vi "MapColor_makeRamp.vi"(1 "ColorMap\narray IN":u32[](array[numeric])=[0, 196608, 393216, 589824, 786432, 983040, 1179648, 1376256, 1572864, 1769472, 1966080, 2162688, 2359296, 2555904, 2752512, 2949120, 3145728, 3342336, 3538944, 3735552, 3932160, 4128768, 4325376, 4521984, 4718592, 4915200, 5111808, 5308416, 5505024, 5701632, 5898240, 6094848, 6291456, 6488064, 6684672, 6881280, 7077888, 7274496, 7471104, 7667712, 7864320, 8060928, 8257536, 8454144, 8650752, 8847360, 9043968, 9240576, 9437184, 9633792, 9830400, 10027008, 10223616, 10420224, 10616832, 10813440, 11010048, 11206656, 11403264, 11599872, 11796480, 11993088, 12189696, 12386304, 12582912, 12779520, 12976128, 13172736, 13369344, 13565952, 13762560, 13959168, 14155776, 14352384, 14548992, 14745600, 14942208, 15138816, 15335424, 15532032, 15728640, 15925248, 16121856, 16318464, 16515072, 16711680, 16712448, 16713216, 16713984, 16714752, 16715520, 16716288, 16717056, 16717824, 16718592, 16719360, 16720128, 16720896, 16721664, 16722432, 16723200, 16723968, 16724736, 16725504, 16726272, 16727040, 16727808, 16728576, 16729344, 16730112, 16730880, 16731648, 16732416, 16733184, 16733952, 16734720, 16735488, 16736256, 16737024, 16737792, 16738560, 16739328, 16740096, 16740864, 16741632, 16742400, 16743168, 16743936, 16744704, 16745472, 16746240, 16747008, 16747776, 16748544, 16749312, 16750080, 16750848, 16751616, 16752384, 16753152, 16753920, 16754688, 16755456, 16756224, 16756992, 16757760, 16758528, 16759296, 16760064, 16760832, 16761600, 16762368, 16763136, 16763904, 16764672, 16765440, 16766208, 16766976, 16767744, 16768512, 16769280, 16770048, 16770816, 16771584, 16772352, 16773120, 16773888, 16774656, 16775424, 16776192, 16776960, 16776963, 16776966, 16776969, 16776972, 16776975, 16776977, 16776980, 16776983, 16776986, 16776989, 16776992, 16776995, 16776998, 16777001, 16777004, 16777007, 16777009, 16777012, 16777015, 16777018, 16777021, 16777024, 16777027, 16777030, 16777033, 16777036, 16777038, 16777041, 16777044, 16777047, 16777050, 16777053, 16777056, 16777059, 16777062, 16777065, 16777068, 16777070, 16777073, 16777076, 16777079, 16777082, 16777085, 16777088, 16777091, 16777094, 16777097, 16777100, 16777102, 16777105, 16777108, 16777111, 16777114, 16777117, 16777120, 16777123, 16777126, 16777129, 16777132, 16777134, 16777137, 16777140, 16777143, 16777146, 16777149, 16777152, 16777155, 16777158, 16777161, 16777163, 16777166, 16777169, 16777172, 16777175, 16777178, 16777181, 16777184, 16777187, 16777190, 16777193, 16777195, 16777198, 16777201, 16777204, 16777207]) -> (0 "ColorMap\narray OUT":u32[](array[numeric])=[0, 196608, 393216, 589824, 786432, 983040, 1179648, 1376256, 1572864, 1769472, 1966080, 2162688, 2359296, 2555904, 2752512, 2949120, 3145728, 3342336, 3538944, 3735552, 3932160, 4128768, 4325376, 4521984, 4718592, 4915200, 5111808, 5308416, 5505024, 5701632, 5898240, 6094848, 6291456, 6488064, 6684672, 6881280, 7077888, 7274496, 7471104, 7667712, 7864320, 8060928, 8257536, 8454144, 8650752, 8847360, 9043968, 9240576, 9437184, 9633792, 9830400, 10027008, 10223616, 10420224, 10616832, 10813440, 11010048, 11206656, 11403264, 11599872, 11796480, 11993088, 12189696, 12386304, 12582912, 12779520, 12976128, 13172736, 13369344, 13565952, 13762560, 13959168, 14155776, 14352384, 14548992, 14745600, 14942208, 15138816, 15335424, 15532032, 15728640, 15925248, 16121856, 16318464, 16515072, 16711680, 16712448, 16713216, 16713984, 16714752, 16715520, 16716288, 16717056, 16717824, 16718592, 16719360, 16720128, 16720896, 16721664, 16722432, 16723200, 16723968, 16724736, 16725504, 16726272, 16727040, 16727808, 16728576, 16729344, 16730112, 16730880, 16731648, 16732416, 16733184, 16733952, 16734720, 16735488, 16736256, 16737024, 16737792, 16738560, 16739328, 16740096, 16740864, 16741632, 16742400, 16743168, 16743936, 16744704, 16745472, 16746240, 16747008, 16747776, 16748544, 16749312, 16750080, 16750848, 16751616, 16752384, 16753152, 16753920, 16754688, 16755456, 16756224, 16756992, 16757760, 16758528, 16759296, 16760064, 16760832, 16761600, 16762368, 16763136, 16763904, 16764672, 16765440, 16766208, 16766976, 16767744, 16768512, 16769280, 16770048, 16770816, 16771584, 16772352, 16773120, 16773888, 16774656, 16775424, 16776192, 16776960, 16776963, 16776966, 16776969, 16776972, 16776975, 16776977, 16776980, 16776983, 16776986, 16776989, 16776992, 16776995, 16776998, 16777001, 16777004, 16777007, 16777009, 16777012, 16777015, 16777018, 16777021, 16777024, 16777027, 16777030, 16777033, 16777036, 16777038, 16777041, 16777044, 16777047, 16777050, 16777053, 16777056, 16777059, 16777062, 16777065, 16777068, 16777070, 16777073, 16777076, 16777079, 16777082, 16777085, 16777088, 16777091, 16777094, 16777097, 16777100, 16777102, 16777105, 16777108, 16777111, 16777114, 16777117, 16777120, 16777123, 16777126, 16777129, 16777132, 16777134, 16777137, 16777140, 16777143, 16777146, 16777149, 16777152, 16777155, 16777158, 16777161, 16777163, 16777166, 16777169, 16777172, 16777175, 16777178, 16777181, 16777184, 16777187, 16777190, 16777193, 16777195, 16777198, 16777201, 16777204, 16777207])   [LabVIEW 2010]
panel:
  in  "ColorMap\nring":u16(ring) caption="Standard Colormap" items=["", "Black-Red-Yellow-White"]
  in  "Cancel":bool
  in  "Accept":bool
  out "VI ref":refnum<vi>
  in  "close":bool
  in  "Scrollbar":i32(c297)=64
  out "ColorRamp":u32[](array[colorbox])=[180, 263349, 526518, 789687, 1052856, 1316026, 1579195, 1842364, 2105533, 2368702, 2631871, 2895040, 3158209, 3421378, 3684548, 3947717, 4145094, 4408263, 4671432, 4934601, 5197770, 5460939, 5724108, 5987278, 6250447, 6513616, 6776785, 7039954, 7303123, 7566292, 7829461, 8092630, 8355800, 8618969, 8882138, 9145307, 9408476, 9671645, 9934814, 10197983, 10461152, 10724322, 10987491, 11250660, 11513829, 11776998, 12040167, 12303336, 12500713, 12763882, 13027052, 13290221, 13553390, 13816559, 14079728, 14342897, 14606066, 14869235, 15132404, 15395574, 15658743, 15921912, 16185081, 16448250, 16448250, 16447222, 16446194, 16445166, 16444138, 16443110, 16442082, 16506590, 16505562, 16504534, 16503506, 16502478, 16501450, 16500422, 16499394, 16498366, 16497595, 16496567, 16495539, 16560047, 16559019, 16557991, 16556963, 16555935, 16554907, 16553879, 16552851, 16551823, 16550795, 16549767, 16548739, 16547711, 16612219, 16611191, 16610163, 16609135, 16608107, 16607079, 16606051, 16605023, 16603995, 16602967, 16601939, 16600911, 16599883, 16664391, 16663363, 16662335, 16661564, 16660536, 16659508, 16658480, 16657452, 16656424, 16655396, 16654368, 16653340, 16717848, 16716820, 16715792, 16714764, 16713736, 16712708, 16711680] caption="Color Ramp"
  out "ColorMap\narray":u32[](array[numeric])=[180, 263349, 526518, 789687, 1052856, 1316026, 1579195, 1842364, 2105533, 2368702, 2631871, 2895040, 3158209, 3421378, 3684548, 3947717, 4145094, 4408263, 4671432, 4934601, 5197770, 5460939, 5724108, 5987278, 6250447, 6513616, 6776785, 7039954, 7303123, 7566292, 7829461, 8092630, 8355800, 8618969, 8882138, 9145307, 9408476, 9671645, 9934814, 10197983, 10461152, 10724322, 10987491, 11250660, 11513829, 11776998, 12040167, 12303336, 12500713, 12763882, 13027052, 13290221, 13553390, 13816559, 14079728, 14342897, 14606066, 14869235, 15132404, 15395574, 15658743, 15921912, 16185081, 16448250, 16448250, 16447993, 16447479, 16447222, 16446965, 16446451, 16446194, 16445937, 16445680, 16445166, 16444909, 16444652, 16444138, 16443881, 16443624, 16443110, 16442853, 16442596, 16442082, 16441825, 16507104, 16506847, 16506333, 16506076, 16505819, 16505305, 16505048, 16504791, 16504277, 16504020, 16503763, 16503249, 16502992, 16502735, 16502221, 16501964, 16501707, 16501450, 16500936, 16500679, 16500422, 16499908, 16499651, 16499394, 16498880, 16498623, 16498366, 16497852, 16497595, 16497338, 16497081, 16496567, 16496310, 16496053, 16495539, 16495282, 16495025, 16494511, 16559790, 16559533, 16559019, 16558762, 16558505, 16558248, 16557734, 16557477, 16557220, 16556706, 16556449, 16556192, 16555678, 16555421, 16555164, 16554650, 16554393, 16554136, 16553879, 16553365, 16553108, 16552851, 16552337, 16552080, 16551823, 16551309, 16551052, 16550795, 16550281, 16550024, 16549767, 16549510, 16548996, 16548739, 16548482, 16547968, 16547711, 16547454, 16612476, 16612219, 16611962, 16611448, 16611191, 16610934, 16610420, 16610163, 16609906, 16609649, 16609135, 16608878, 16608621, 16608107, 16607850, 16607593, 16607079, 16606822, 16606565, 16606051, 16605794, 16605537, 16605280, 16604766, 16604509, 16604252, 16603738, 16603481, 16603224, 16602710, 16602453, 16602196, 16601682, 16601425, 16601168, 16600911, 16600397, 16600140, 16665419, 16664905, 16664648, 16664391, 16663877, 16663620, 16663363, 16662849, 16662592, 16662335, 16662078, 16661564, 16661307, 16661050, 16660536, 16660279, 16660022, 16659508, 16659251, 16658994, 16658480, 16658223, 16657966, 16657709, 16657195, 16656938, 16656681, 16656167, 16655910, 16655653, 16655139, 16654882, 16654625, 16654111, 16653854, 16653597, 16653083, 16652826, 16718105, 16717848, 16717334, 16717077, 16716820, 16716306, 16716049, 16715792, 16715278, 16715021, 16714764, 16714250, 16713993, 16713736, 16713479, 16712965, 16712708, 16712451, 16711937, 16711680]
  in  "Color 3":u32(colorbox)=16711680
  in  "Color 2":u32(colorbox)=16448250
  in  "Color 1":u32(colorbox)=180
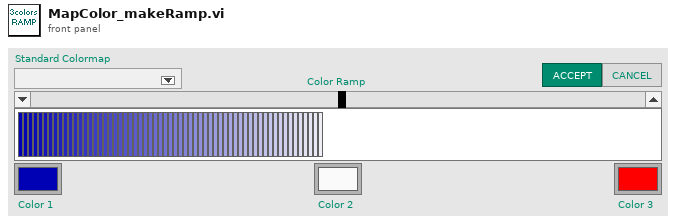
[diagram p1: front panel]
types:
  T1 = enum32{"Invalid", "Standard", "Closed", "Hidden", "Minimized", "Maximized"}
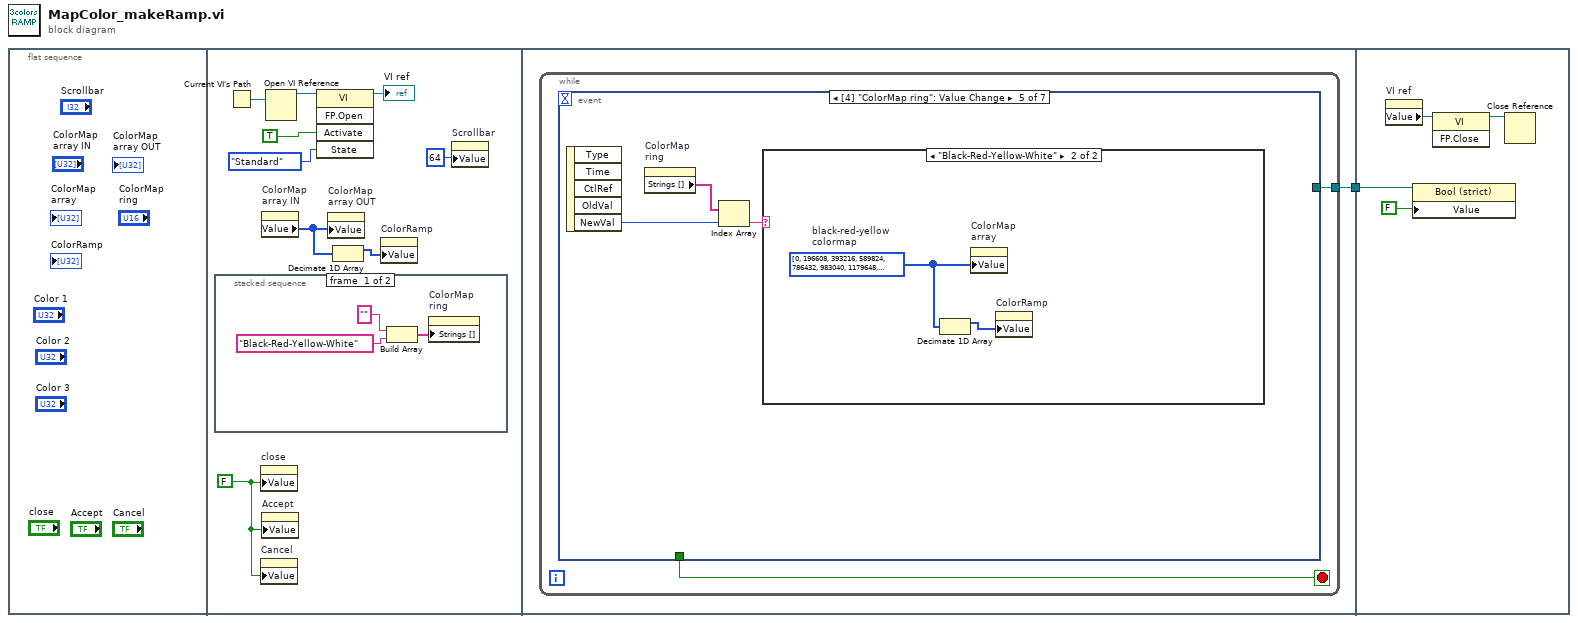
[diagram p0: block diagram]
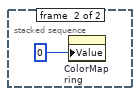
[diagram p2: hidden frame]
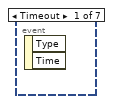
[diagram p3: hidden frame]
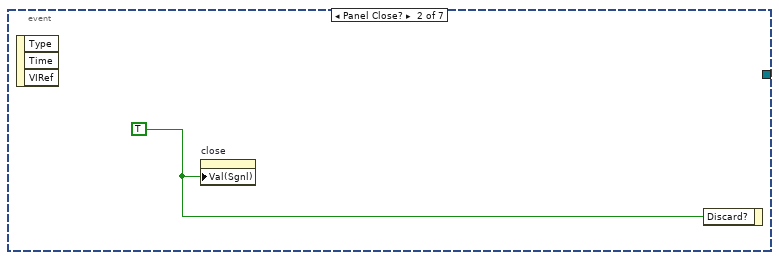
[diagram p4: hidden frame]
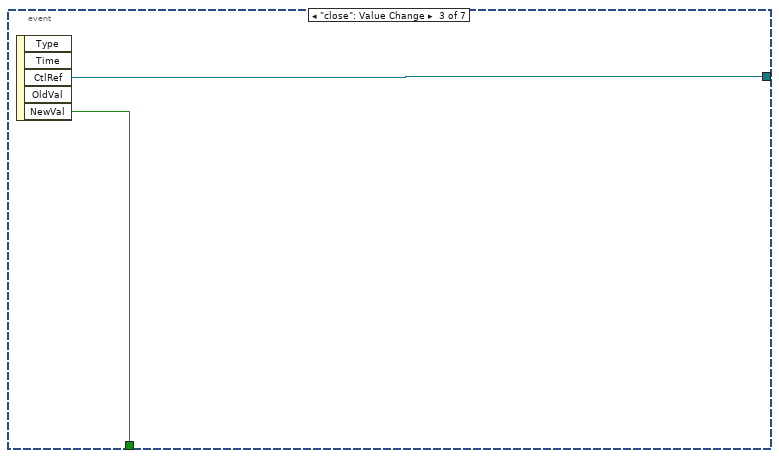
[diagram p5: hidden frame]
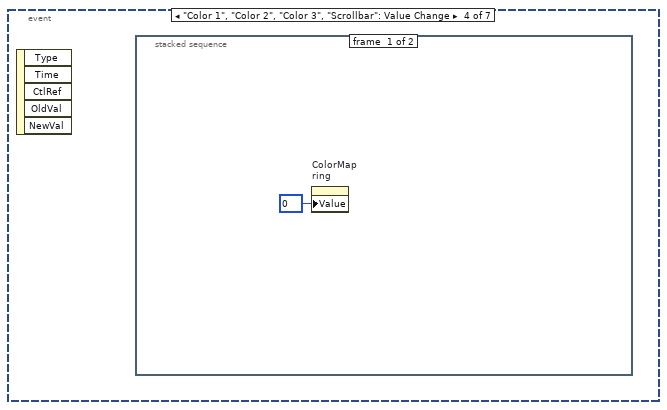
[diagram p6: hidden frame]
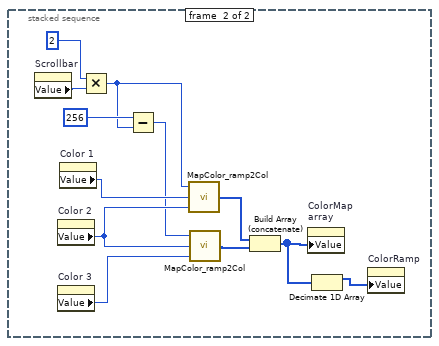
[diagram p7: hidden frame]
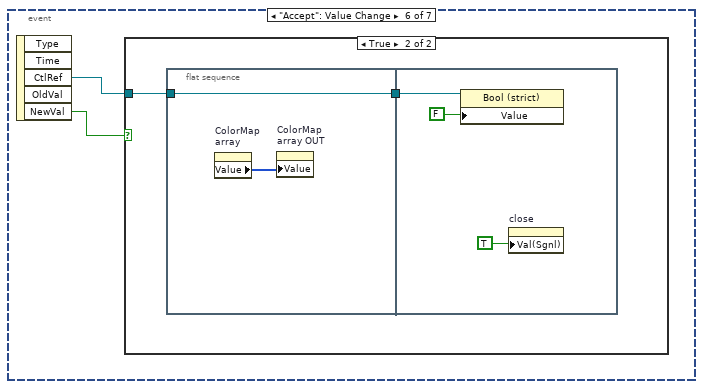
[diagram p9: hidden frame]
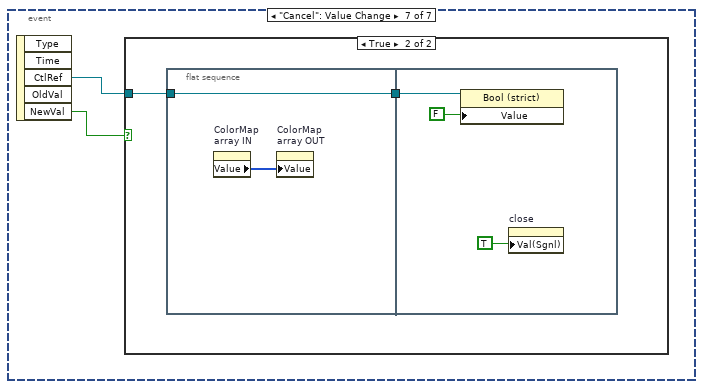
[diagram p11: hidden frame]
diagram:
  n1 = flat-sequence {
    tunnel: [w15] -> w1
    tunnel: w1 -> [w60]
    frame #0 {
    }
    frame #1 {
      w4 = FALSE ("close")
      n2 = stacked-sequence {
        frame #0 {
          n3 = Build Array("" ("element"), "Black-Red-Yellow-White") -> (w12:string[])
          n4 = property on="ColorMap\nring" class="Ring (strict)"("Strings []"=w12) -> ()  [unwired: 2 in, 2 out]
        }
        frame #1 {
          n5 = property on="ColorMap\nring" class="Ring (strict)"("Value"=0) -> ()  [unwired: 2 in, 2 out]
        }
      }
      n6 = Current VI's Path() -> (path=w9:path)
      n7 = property on="close" class="Bool (strict)"("Value"=w4) -> ()  [unwired: 2 in, 2 out]
      n8 = property on="Cancel" class="Bool (strict)"("Value"=w4) -> ()  [unwired: 2 in, 2 out]
      n9 = property on="ColorMap\narray IN" class="Arr (strict)"() -> ("Value"=w3:u32[])  [unwired: 2 in, 2 out]
      n10 = property on="Accept" class="Bool (strict)"("Value"=w4) -> ()  [unwired: 2 in, 2 out]
      n11 = Open VI Reference(vi path=w9) -> (vi reference=w8:refnum<vi>)  [unwired: 5 in, 1 out]
      n12 = invoke class="VI" method="FP.Open"(reference=w8, "Activate"=TRUE ("Activate?"), "State"=T1."Standard") -> (reference out=→"VI ref":refnum<vi>)  [unwired: 2 in, 4 out]
      n13 = property on="ColorMap\narray OUT" class="Arr (strict)"("Value"=w3) -> ()  [unwired: 2 in, 2 out]
      n14 = Decimate 1D Array(w3) -> (w2:u32[])  [unwired: 1 out]
      n15 = property on="ColorRamp" class="Arr (strict)"("Value"=w2) -> ()  [unwired: 2 in, 2 out]
      n16 = property on="Scrollbar" class="Scroll (strict)"("Value"=64 ("Scrollbar")) -> ()  [unwired: 2 in, 2 out]
    }
    frame #2 {
      n17 = while {
        tunnel: [w16] -> w15
        stop <- w17 stop-if-true
        n18 = event shown="[4] \"ColorMap\nring\": Value Change" {
          selector: _ -> [_ _ _ _ _ _ _]
          dyn-events: _ -> [_ _ _ _ _ _ _]
          timeout: _ -> [_ _ _ _ _ _ _]
          tunnel: [_ _ w20 _ _ _ _] -> w17
          tunnel: [_ _ w19 _ _ _ _] -> w16
          event Timeout {
            n19 = event-data() -> ()  [unwired: 1 in, 2 out]
          }
          event Panel Close? {
            w18 = TRUE
            n20 = event-data() -> ()  [unwired: 1 in, 3 out]
            n21 = property on="close" class="Bool (strict)"("Val(Sgnl)"=w18) -> ()  [unwired: 2 in, 2 out]
            n22 = event-data("Discard?"=w18) -> ()  [unwired: 1 in, 1 out]
          }
          event "close": Value Change {
            n23 = event-data() -> ("CtlRef"=w19:refnum<vi>, "NewVal"=w20:bool)  [unwired: 1 in, 3 out]
          }
          event "Color 1", "Color 2", "Color 3", "Scrollbar": Value Change {
            n24 = event-data() -> ()  [unwired: 1 in, 5 out]
            n25 = stacked-sequence {
              frame #0 {
                w21 = u16 0 items=["", "Black-red-yellow"] ("ColorMap\nring")
                n26 = property on="ColorMap\nring" class="Ring (strict)"("Value"=w21) -> ()  [unwired: 2 in, 2 out]
              }
              frame #1 {
                n27 = property on="Scrollbar" class="Scroll (strict)"() -> ("Value"=w26:i32)  [unwired: 2 in, 2 out]
                n28 = property on="Color 2" class="ColBox"() -> ("Value"=w30:u32)  [unwired: 2 in, 2 out]
                n29 = property on="Color 3" class="ColBox"() -> ("Value"=w29:u32)  [unwired: 2 in, 2 out]
                n30 = property on="Color 1" class="ColBox"() -> ("Value"=w31:u32)  [unwired: 2 in, 2 out]
                n31 = Multiply(x=2, y=w26) -> (x*y=w25:i32)
                n32 = Subtract(x=256, y=w25) -> (x-y=w27:i32)
                n33 = call "MapColor_ramp2Col.vi"("Color 2"=w30, "Color 1"=w31, "numColors"=w25) -> ("appended array"=w33:u32[])
                n34 = call "MapColor_ramp2Col.vi"("Color 2"=w29, "Color 1"=w30, "numColors"=w27) -> ("appended array"=w32:u32[])
                n35 = Build Array (concatenate)(w33, w32) -> (w22:u32[])
                n36 = property on="ColorMap\narray" class="Arr (strict)"("Value"=w22) -> ()  [unwired: 2 in, 2 out]
                n37 = Decimate 1D Array(w22) -> (w23:u32[])  [unwired: 1 out]
                n38 = property on="ColorRamp" class="Arr (strict)"("Value"=w23) -> ()  [unwired: 2 in, 2 out]
              }
            }
          }
          event "ColorMap\nring": Value Change {
            n39 = event-data() -> ("NewVal"=w35:u16)  [unwired: 1 in, 4 out]
            n40 = property on="ColorMap\nring" class="Ring (strict)"() -> ("Strings []"=w36:string[])  [unwired: 2 in, 2 out]
            n41 = Index Array(array=w36, index=w35) -> (element=w34:string)
            n42 = case shown="\"Black-Red-Yellow-White\"" w34 {
              frame Default {
              }
              frame "Black-Red-Yellow-White" {
                w38 = u32[] [0, 196608, 393216, 589824, 786432, 983040, 1179648, 1376256, 1572864, 1769472, 1966080, 2162688, 2359296, 2555904, 2752512, 2949120, 3145728, 3342336, 3538944, 3735552, 3932160, 4128768, 4325376, 4521984, 4718592, 4915200, 5111808, 5308416, 5505024, 5701632, 5898240, 6094848, 6291456, 6488064, 6684672, 6881280, 7077888, 7274496, 7471104, 7667712, 7864320, 8060928, 8257536, 8454144, 8650752, 8847360, 9043968, 9240576, 9437184, 9633792, 9830400, 10027008, 10223616, 10420224, 10616832, 10813440, 11010048, 11206656, 11403264, 11599872, 11796480, 11993088, 12189696, 12386304, 12582912, 12779520, 12976128, 13172736, 13369344, 13565952, 13762560, 13959168, 14155776, 14352384, 14548992, 14745600, 14942208, 15138816, 15335424, 15532032, 15728640, 15925248, 16121856, 16318464, 16515072, 16711680, 16712448, 16713216, 16713984, 16714752, 16715520, 16716288, 16717056, 16717824, 16718592, 16719360, 16720128, 16720896, 16721664, 16722432, 16723200, 16723968, 16724736, 16725504, 16726272, 16727040, 16727808, 16728576, 16729344, 16730112, 16730880, 16731648, 16732416, 16733184, 16733952, 16734720, 16735488, 16736256, 16737024, 16737792, 16738560, 16739328, 16740096, 16740864, 16741632, 16742400, 16743168, 16743936, 16744704, 16745472, 16746240, 16747008, 16747776, 16748544, 16749312, 16750080, 16750848, 16751616, 16752384, 16753152, 16753920, 16754688, 16755456, 16756224, 16756992, 16757760, 16758528, 16759296, 16760064, 16760832, 16761600, 16762368, 16763136, 16763904, 16764672, 16765440, 16766208, 16766976, 16767744, 16768512, 16769280, 16770048, 16770816, 16771584, 16772352, 16773120, 16773888, 16774656, 16775424, 16776192, 16776960, 16776963, 16776966, 16776969, 16776972, 16776975, 16776977, 16776980, 16776983, 16776986, 16776989, 16776992, 16776995, 16776998, 16777001, 16777004, 16777007, 16777009, 16777012, 16777015, 16777018, 16777021, 16777024, 16777027, 16777030, 16777033, 16777036, 16777038, 16777041, 16777044, 16777047, 16777050, 16777053, 16777056, 16777059, 16777062, 16777065, 16777068, 16777070, 16777073, 16777076, 16777079, 16777082, 16777085, 16777088, 16777091, 16777094, 16777097, 16777100, 16777102, 16777105, 16777108, 16777111, 16777114, 16777117, 16777120, 16777123, 16777126, 16777129, 16777132, 16777134, 16777137, 16777140, 16777143, 16777146, 16777149, 16777152, 16777155, 16777158, 16777161, 16777163, 16777166, 16777169, 16777172, 16777175, 16777178, 16777181, 16777184, 16777187, 16777190, 16777193, 16777195, 16777198, 16777201, 16777204, 16777207]  # black-red-yellow colormap
                n43 = Decimate 1D Array(w38) -> (w37:u32[])  [unwired: 1 out]
                n44 = property on="ColorMap\narray" class="Arr (strict)"("Value"=w38) -> ()  [unwired: 2 in, 2 out]
                n45 = property on="ColorRamp" class="Arr (strict)"("Value"=w37) -> ()  [unwired: 2 in, 2 out]
              }
            }
          }
          event "Accept": Value Change {
            n46 = event-data() -> ("CtlRef"=w39:refnum<vi>, "NewVal"=w40:bool)  [unwired: 1 in, 3 out]
            n47 = case shown="True" w40 {
              tunnel: w39 -> [_ w41]
              frame False {
              }
              frame True {
                n48 = flat-sequence {
                  tunnel: [w43] -> w42
                  tunnel: w41 -> [w43]
                  tunnel: w42 -> [w46]
                  frame #0 {
                    n49 = property on="ColorMap\narray" class="Arr (strict)"() -> ("Value"=w44:u32[])  [unwired: 2 in, 2 out]
                    n50 = property on="ColorMap\narray OUT" class="Arr (strict)"("Value"=w44) -> ()  [unwired: 2 in, 2 out]
                  }
                  frame #1 {
                    n51 = property class="Bool (strict)"(reference=w46, "Value"=FALSE) -> ()  [unwired: 1 in, 2 out]
                    n52 = property on="close" class="Bool (strict)"("Val(Sgnl)"=TRUE ("Value (Signaling)")) -> ()  [unwired: 2 in, 2 out]
                  }
                }
              }
            }
          }
          event "Cancel": Value Change {
            n53 = event-data() -> ("CtlRef"=w48:refnum<vi>, "NewVal"=w49:bool)  [unwired: 1 in, 3 out]
            n54 = case shown="True" w49 {
              tunnel: w48 -> [_ w50]
              frame False {
              }
              frame True {
                n55 = flat-sequence {
                  tunnel: [w53] -> w51
                  tunnel: w50 -> [w53]
                  tunnel: w51 -> [w55]
                  frame #0 {
                    n56 = property on="ColorMap\narray IN" class="Arr (strict)"() -> ("Value"=w52:u32[])  [unwired: 2 in, 2 out]
                    n57 = property on="ColorMap\narray OUT" class="Arr (strict)"("Value"=w52) -> ()  [unwired: 2 in, 2 out]
                  }
                  frame #1 {
                    n58 = property class="Bool (strict)"(reference=w55, "Value"=FALSE) -> ()  [unwired: 1 in, 2 out]
                    n59 = property on="close" class="Bool (strict)"("Val(Sgnl)"=TRUE ("Value (Signaling)")) -> ()  [unwired: 2 in, 2 out]
                  }
                }
              }
            }
          }
        }
      }
    }
    frame #3 {
      n60 = property on="VI ref" class="VIRef (strict)"() -> ("Value"=w58:refnum<vi>)  [unwired: 2 in, 2 out]
      n61 = property class="Bool (strict)"(reference=w60, "Value"=FALSE) -> ()  [unwired: 1 in, 2 out]
      n62 = invoke class="VI" method="FP.Close"(reference=w58) -> (reference out=w57:refnum<vi>)  [unwired: 2 in, 2 out]
      n63 = Close Reference(reference=w57) -> ()  [unwired: 1 in, 1 out]
    }
  }
